vi "HFRR ADV v06.vi"() -> ()   [LabVIEW 2025] (continued)
                  n3132 = property on="Sample Temperature ( °C )" class="XYGraph (strict)"("X Scale.Name Label.Text"=w4406) -> ()  [unwired: 2 in, 2 out]
                  n3133 = property on="Coefficient Of Friction" class="XYGraph (strict)"("X Scale.Name Label.Text"=w4406) -> ()  [unwired: 2 in, 2 out]
                }
                frame 81 {
                  n3134 = property on="Air Temperature  ( °C )" class="XYGraph (strict)"("Y Scale.Name Label.Text"=w4407) -> ()  [unwired: 2 in, 2 out]
                }
                frame 82 {
                  n3135 = local write "S 84"(w4408) -> ()
                }
                frame 83 {
                  n3136 = local write "S 85"(w4409) -> ()
                }
                frame 84 {
                  n3137 = local write "S 86"(w4410) -> ()
                }
                frame 85 {
                  n3138 = local write "S 87"(w4411) -> ()
                }
                frame 86 {
                  n3139 = local write "S 88"(w4412) -> ()
                }
                frame 87 {
                  n3140 = property on="FF Calibration g" class="WFGraph (strict)"("Y Scale.Name Label.Text"=w4413) -> ()  [unwired: 2 in, 2 out]
                }
                frame 88 {
                  n3141 = local write "S 90"(w4414) -> ()
                }
                frame 89 {
                  n3142 = local write "S 91"(w4415) -> ()
                }
                frame 90 {
                  n3143 = local write "S 92"(w4416) -> ()
                }
                frame 91 {
                  n3144 = local write "S 93"(w4417) -> ()
                }
                frame 92 {
                  n3145 = local write "S 94"(w4418) -> ()
                }
                frame 93 {
                  n3146 = local write "S 95"(w4419) -> ()
                }
                frame 94 {
                  n3147 = local write "S 96"(w4420) -> ()
                }
                frame 95 {
                  n3148 = local write "S 97"(w4421) -> ()
                }
                frame 96 {
                  n3149 = local write "S 98"(w4422) -> ()
                }
                frame 97 {
                  n3150 = local write "S 99"(w4423) -> ()
                }
                frame 98 {
                  n3151 = local write "S 100"(w4424) -> ()
                }
                frame 99 {
                  n3152 = local write "S 101"(w4425) -> ()
                }
                frame 100 {
                  n3153 = local write "S 102"(w4426) -> ()
                }
                frame 101 {
                  n3154 = local write "S 103"(w4427) -> ()
                }
                frame 102 {
                  n3155 = local write "S 104"(w4428) -> ()
                }
                frame 103 {
                  n3156 = local write "S 105"(w4429) -> ()
                }
                frame 104 {
                  n3157 = local write "S 106"(w4430) -> ()
                }
                frame 105 {
                }
                frame 106 {
                  n3158 = property on="OK Button 17" class="Bool (strict)"("Boolean Text.Text"=w4431) -> ()  [unwired: 2 in, 2 out]
                }
                frame 107 {
                  n3159 = property on="OK Button 16" class="Bool (strict)"("Boolean Text.Text"=w4432) -> ()  [unwired: 2 in, 2 out]
                }
                frame 108 {
                  n3160 = property on="TITTLE" class="Str"("Caption.Text"=w4433) -> ()  [unwired: 2 in, 2 out]
                }
                frame 109 {
                  "String 30" <- w4434
                }
                frame 110 {
                  n3161 = property on="Test Date" class="Str"("Caption.Text"=w4435) -> ()  [unwired: 2 in, 2 out]
                  "String 31" <- w4435
                }
                frame 111 {
                  n3162 = property on="Sample ID" class="Str"("Caption.Text"=w4436) -> ()  [unwired: 2 in, 2 out]
                  "String 32" <- w4436
                }
                frame 112 {
                  n3163 = property on="Tested by" class="Str"("Caption.Text"=w4437) -> ()  [unwired: 2 in, 2 out]
                  "String 33" <- w4437
                }
                frame 113 {
                  n3164 = property on="System Configured Printers 2" class="Arr (strict)"("Caption.Text"=w4438) -> ()  [unwired: 2 in, 2 out]
                }
                frame 114 {
                  n3165 = property on="Selected Printer" class="Str"("Caption.Text"=w4439) -> ()  [unwired: 2 in, 2 out]
                }
                frame 115 {
                  n3166 = property on="Select Printer 3" class="DigNum (strict)"("Caption.Text"=w4440) -> ()  [unwired: 2 in, 2 out]
                }
                frame 116 {
                  n3167 = property on="Print" class="Bool (strict)"("Boolean Text.Text"=w4441) -> ()  [unwired: 2 in, 2 out]
                }
                frame 117 {
                  "String 41" <- w4442
                }
                frame 118 {
                  n3168 = property on="tested by" class="Str"("Caption.Text"=w4443) -> ()  [unwired: 2 in, 2 out]
                }
                frame 119 {
                }
                frame 120 {
                  n3169 = property on="Export" class="Bool (strict)"("Boolean Text.Text"=w4444) -> ()  [unwired: 2 in, 2 out]
                }
                frame 121 {
                  n3170 = property on="TEMP INTERCEPT:" class="DigNum (strict)"("Caption.Text"=w4445) -> ()  [unwired: 2 in, 2 out]
                }
                frame 122 {
                  n3171 = property on="AIR TEMP INTERCEPT:" class="DigNum (strict)"("Caption.Text"=w4446) -> ()  [unwired: 2 in, 2 out]
                }
                frame 123 {
                  n3172 = property on="Select File Type" class="Enum (strict)"("Caption.Text"=w4447) -> ()  [unwired: 2 in, 2 out]
                }
                frame 124 {
                  n3173 = property on="s.NO" class="Str"("Caption.Text"=w4448) -> ()  [unwired: 2 in, 2 out]
                  "String 45" <- w4448
                }
                frame 125 {
                  n3174 = property on="trip1 8" class="Bool (strict)"("Boolean Text.Text"=w4449) -> ()  [unwired: 2 in, 2 out]
                }
                frame 126, Default {
                }
              }
            }
          }
          frame #1 {
            w4457 = TRUE ("Visible")
            n3175 = local read "S 91"() -> (w4474:string)
            n3176 = local read "S 90"() -> (w4473:string)
            n3177 = local read "S 88"() -> (w4472:string)
            n3178 = property on="Threshold" class="DigNum (strict)"("Caption.Text"=w4474) -> ()  [unwired: 2 in, 2 out]
            n3179 = property on="File Path" class="Path"("Caption.Text"=w4473) -> ()  [unwired: 2 in, 2 out]
            n3180 = property on="SrvM CP" class="Bool (strict)"("Boolean Text.Text"=w4472) -> ()  [unwired: 2 in, 2 out]
            n3181 = local read "S 71"() -> (w4467:string)
            n3182 = local read "S 86"() -> (w4469:string)
            n3183 = local read "S 85"() -> (w4470:string)
            n3184 = local read "S 87"() -> (w4468:string)
            n3185 = local read "S 84"() -> (w4471:string)
            n3186 = local read "S 103"() -> (w4456:string)
            n3187 = local read "S 104"() -> (w4455:string)
            n3188 = property on="ENTER THE NEW PASSWORD" class="Str"("Caption.Text"=w4468) -> ()  [unwired: 2 in, 2 out]
            n3189 = property on="Password" class="Str"("Caption.Text"=w4470) -> ()  [unwired: 2 in, 2 out]
            n3190 = property on="ENTER CURRENT PASSWORD" class="Str"("Caption.Text"=w4469) -> ()  [unwired: 2 in, 2 out]
            n3191 = property on="EDIT" class="Bool (strict)"("Boolean Text.Text"=w4467) -> ()  [unwired: 2 in, 2 out]
            n3192 = property on="SAVE" class="Bool (strict)"("Boolean Text.Text"=w4471) -> ()  [unwired: 2 in, 2 out]
            n3193 = Build Array(w4456, w4455) -> (w4454:string[])
            n3194 = property on="Heater Button" class="Bool (strict)"("Strings [4]"=w4454) -> ()  [unwired: 2 in, 2 out]
            n3195 = property on="CH-HUMIDITY WET" class="DigNum (strict)"("Caption.Size to Text?"=w4457) -> ()  [unwired: 2 in, 2 out]
            n3196 = property on="CH-HUMIDITY DRY" class="DigNum (strict)"("Caption.Size to Text?"=w4457) -> ()  [unwired: 2 in, 2 out]
            n3197 = property on="CH-POWER -" class="DigNum (strict)"("Caption.Size to Text?"=w4457) -> ()  [unwired: 2 in, 2 out]
            n3198 = property on="CH-HEATER" class="DigNum (strict)"("Caption.Size to Text?"=w4457) -> ()  [unwired: 2 in, 2 out]
            n3199 = property on="CH-POWER +" class="DigNum (strict)"("Caption.Size to Text?"=w4457) -> ()  [unwired: 2 in, 2 out]
            n3200 = local read "S 92"() -> (w4466:string)
            n3201 = local read "S 93"() -> (w4465:string)
            n3202 = local read "S 105"() -> (w4452:string)
            n3203 = local read "S 106"() -> (w4451:string)
            n3204 = Build Array(w4466, w4465) -> ()  [unwired: 1 out]
            n3205 = Build Array(w4452, w4451) -> (w4453:string[])
            n3206 = local read "S 95"() -> (w4463:string)
            n3207 = local read "S 94"() -> (w4464:string)
            n3208 = local read "bs"() -> (w4479:string)
            n3209 = local read "as"() -> (w4480:string)
            n3210 = property on="Humidity" class="Bool (strict)"("Strings [4]"=w4453) -> ()  [unwired: 2 in, 2 out]
            n3211 = Concatenate Strings(w4479, "\r", w4480) -> ()  [unwired: 1 out]
            n3212 = property on="STROKE GAIN :" class="DigNum (strict)"("Caption.Text"=w4463) -> ()  [unwired: 2 in, 2 out]
            n3213 = property on="DISPLACEMENT :" class="DigNum (strict)"("Caption.Text"=w4464) -> ()  [unwired: 2 in, 2 out]
            n3214 = property on="Rh After" class="DigNum (strict)"("Caption.Size to Text?"=TRUE ("Caption.Size to Text")) -> ()  [unwired: 2 in, 2 out]
            n3215 = local read "S 48"() -> (w4503:string)
            n3216 = local read "S 50"() -> (w4501:string)
            n3217 = local read "S 51"() -> (w4500:string)
            n3218 = local read "S 49"() -> (w4502:string)
            n3219 = local read "S 52"() -> (w4499:string)
            n3220 = local read "as"() -> (w4484:string)
            n3221 = local read "bs"() -> (w4485:string)
            n3222 = local read "S 56"() -> (w4498:string)
            n3223 = local read "S 57"() -> (w4497:string)
            n3224 = local read "S 58"() -> (w4496:string)
            n3225 = local read "S 59"() -> (w4495:string)
            n3226 = property on="OPEN" class="Bool (strict)"("Boolean Text.Text"=w4499) -> ()  [unwired: 2 in, 2 out]
            n3227 = property on="OPEN 1" class="Bool (strict)"("Boolean Text.Text"=w4503) -> ()  [unwired: 2 in, 2 out]
            n3228 = property on="OPEN 2" class="Bool (strict)"("Boolean Text.Text"=w4502) -> ()  [unwired: 2 in, 2 out]
            n3229 = property on="OPEN 3" class="Bool (strict)"("Boolean Text.Text"=w4501) -> ()  [unwired: 2 in, 2 out]
            n3230 = property on="OPEN 4" class="Bool (strict)"("Boolean Text.Text"=w4500) -> ()  [unwired: 2 in, 2 out]
            n3231 = Concatenate Strings(w4485, "\r", w4484) -> ()  [unwired: 1 out]
            n3232 = local read "S 102"() -> (w4458:string)
            n3233 = property on="КОФ1" class="DigNum (strict)"("Caption.Text"=w4498) -> ()  [unwired: 2 in, 2 out]
            n3234 = local read "S 98"() -> (w4462:string)
            n3235 = local read "S 99"() -> (w4461:string)
            n3236 = local read "S 100"() -> (w4460:string)
            n3237 = local read "S 101"() -> (w4459:string)
            n3238 = property on="КОФ2" class="DigNum (strict)"("Caption.Text"=w4497) -> ()  [unwired: 2 in, 2 out]
            n3239 = property on="КОФ3" class="DigNum (strict)"("Caption.Text"=w4496) -> ()  [unwired: 2 in, 2 out]
            n3240 = property on="КОФ4" class="DigNum (strict)"("Caption.Text"=w4495) -> ()  [unwired: 2 in, 2 out]
            n3241 = local read "bs"() -> (w4483:string)
            n3242 = local read "as"() -> (w4482:string)
            n3243 = property on="CH-POWER +" class="DigNum (strict)"("Caption.Text"=w4462) -> ()  [unwired: 2 in, 2 out]
            n3244 = property on="CH-POWER -" class="DigNum (strict)"("Caption.Text"=w4461) -> ()  [unwired: 2 in, 2 out]
            n3245 = property on="CH-HEATER" class="DigNum (strict)"("Caption.Text"=w4460) -> ()  [unwired: 2 in, 2 out]
            n3246 = property on="CH-HUMIDITY DRY" class="DigNum (strict)"("Caption.Text"=w4459) -> ()  [unwired: 2 in, 2 out]
            n3247 = property on="CH-HUMIDITY WET" class="DigNum (strict)"("Caption.Text"=w4458) -> ()  [unwired: 2 in, 2 out]
            n3248 = local read "S 60"() -> (w4494:string)
            n3249 = local read "S 54"() -> (w4504:string)
            n3250 = Concatenate Strings(w4483, "\r", w4482) -> ()  [unwired: 1 out]
            n3251 = Concatenate Strings(w4504, w4494) -> ()  [unwired: 1 out]
            n3252 = local read "S 77"() -> (→"String 43":string)
            n3253 = local read "S 76"() -> (w4477:string)
            n3254 = local read "S 78"() -> (w4476:string)
            n3255 = local read "S 71"() -> (w4488:string)
            n3256 = local read "S 66"() -> (w4493:string)
            n3257 = local read "S 67"() -> (w4492:string)
            n3258 = local read "S 68"() -> (w4491:string)
            n3259 = local read "S 69"() -> (w4490:string)
            n3260 = local read "S 70"() -> (w4489:string)
            n3261 = property on="AIR TEMP" class="DigNum (strict)"("Caption.Text"=w4476) -> ()  [unwired: 2 in, 2 out]
            n3262 = property on="Set Strk" class="DigNum (strict)"("Caption.Text"=w4477) -> ()  [unwired: 2 in, 2 out]
            n3263 = property on="FRIC. FORCE :" class="DigNum (strict)"("Caption.Text"=w4493) -> ()  [unwired: 2 in, 2 out]
            n3264 = property on="TEMPERATURE :" class="DigNum (strict)"("Caption.Text"=w4492) -> ()  [unwired: 2 in, 2 out]
            n3265 = property on="SPEED OUT:" class="DigNum (strict)"("Caption.Text"=w4491) -> ()  [unwired: 2 in, 2 out]
            n3266 = property on="AIR TEMPERATURE :" class="DigNum (strict)"("Caption.Text"=w4490) -> ()  [unwired: 2 in, 2 out]
            n3267 = property on="HUMIDITY:" class="DigNum (strict)"("Caption.Text"=w4489) -> ()  [unwired: 2 in, 2 out]
            n3268 = property on="EDIT" class="Bool (strict)"("Boolean Text.Text"=w4488) -> ()  [unwired: 2 in, 2 out]
            n3269 = local read "S 79"() -> (w4475:string)
            n3270 = property on="Stroke" class="DigNum (strict)"("Caption.Text"=w4475) -> ()  [unwired: 2 in, 2 out]
          }
          frame #2 {
          }
        }
        n3271 = local write "Lan flag"(10.0 ("Lan flag")) -> ()
      }
      frame Enabled {
      }
    }
    n3272 = Wait (ms)(milliseconds to wait=u32 2000) -> ()  [unwired: 1 out]
    n3273 = local read "Quit"() -> (w4277:bool)
  }
  n3274 = disable-structure shown="Disabled" {
    frame Disabled {
      n3275 = while {
        tunnel: [w4506] -> _
        i -> [w4506]
        stop <- w4505 continue-if-true
        n3276 = Wait (ms)(milliseconds to wait=u32 50) -> ()  [unwired: 1 out]
        n3277 = stacked-sequence {
          frame #0 {
            # "Controls Text color"
            # "Controls BG color"
            n3278 = property on="FILE" class="Str"("Text.Text Colors:Text Color"="SC  Text") -> ()  [unwired: 2 in, 2 out]
            n3279 = property on="Fuel Discription :" class="Str"("Text.Text Colors:Text Color"="SC  Text") -> ()  [unwired: 2 in, 2 out]
            n3280 = property on="tested by" class="Str"("Text.Text Colors:Text Color"="SC  Text") -> ()  [unwired: 2 in, 2 out]
            n3281 = property on="Remarks :" class="Str"("Text.Text Colors:Text Color"="SC  Text") -> ()  [unwired: 2 in, 2 out]
            n3282 = property class="DigNum (strict)"("Numeric Text.Text Colors:BG Color"="NC BG") -> ()  [unwired: 2 in, 2 out]
            n3283 = property class="DigNum (strict)"("Numeric Text.Text Colors:BG Color"="NC BG") -> ()  [unwired: 2 in, 2 out]
            n3284 = property class="DigNum (strict)"("Numeric Text.Text Colors:BG Color"="NC BG") -> ()  [unwired: 2 in, 2 out]
            n3285 = property class="DigNum (strict)"("Numeric Text.Text Colors:BG Color"="NC BG") -> ()  [unwired: 2 in, 2 out]
            n3286 = property class="DigNum (strict)"("Numeric Text.Text Colors:BG Color"="NC BG") -> ()  [unwired: 2 in, 2 out]
            n3287 = property class="DigNum (strict)"("Numeric Text.Text Colors:BG Color"="NC BG") -> ()  [unwired: 2 in, 2 out]
            n3288 = property class="DigNum (strict)"("Numeric Text.Text Colors:BG Color"="NC BG") -> ()  [unwired: 2 in, 2 out]
            n3289 = property class="DigNum (strict)"("Numeric Text.Text Colors:BG Color"="NC BG") -> ()  [unwired: 2 in, 2 out]
            n3290 = property class="DigNum (strict)"("Numeric Text.Text Colors:BG Color"="NC BG") -> ()  [unwired: 2 in, 2 out]
            n3291 = property class="DigNum (strict)"("Numeric Text.Text Colors:BG Color"="NC BG") -> ()  [unwired: 2 in, 2 out]
            n3292 = property class="DigNum (strict)"("Numeric Text.Text Colors:BG Color"="NC BG") -> ()  [unwired: 2 in, 2 out]
            n3293 = property class="DigNum (strict)"("Numeric Text.Text Colors:BG Color"="NC BG") -> ()  [unwired: 2 in, 2 out]
            n3294 = property on="FILE" class="Str"("Text.Text Colors:BG Color"="SC BG 3") -> ()  [unwired: 2 in, 2 out]
            n3295 = property on="Fuel Discription :" class="Str"("Text.Text Colors:BG Color"="SC BG 3") -> ()  [unwired: 2 in, 2 out]
            n3296 = property on="tested by" class="Str"("Text.Text Colors:BG Color"="SC BG 3") -> ()  [unwired: 2 in, 2 out]
            n3297 = property on="Remarks :" class="Str"("Text.Text Colors:BG Color"="SC BG 3") -> ()  [unwired: 2 in, 2 out]
            n3298 = property class="DigNum (strict)"("Numeric Text.Text Colors:Text Color"="NC Text") -> ()  [unwired: 2 in, 2 out]
            n3299 = property class="DigNum (strict)"("Numeric Text.Text Colors:Text Color"="NC Text") -> ()  [unwired: 2 in, 2 out]
            n3300 = property class="DigNum (strict)"("Numeric Text.Text Colors:Text Color"="NC Text") -> ()  [unwired: 2 in, 2 out]
            n3301 = property class="DigNum (strict)"("Numeric Text.Text Colors:Text Color"="NC Text") -> ()  [unwired: 2 in, 2 out]
            n3302 = property class="DigNum (strict)"("Numeric Text.Text Colors:Text Color"="NC Text") -> ()  [unwired: 2 in, 2 out]
            n3303 = property class="DigNum (strict)"("Numeric Text.Text Colors:Text Color"="NC Text") -> ()  [unwired: 2 in, 2 out]
            n3304 = property class="DigNum (strict)"("Numeric Text.Text Colors:Text Color"="NC Text") -> ()  [unwired: 2 in, 2 out]
            n3305 = property class="DigNum (strict)"("Numeric Text.Text Colors:Text Color"="NC Text") -> ()  [unwired: 2 in, 2 out]
            n3306 = property class="DigNum (strict)"("Numeric Text.Text Colors:Text Color"="NC Text") -> ()  [unwired: 2 in, 2 out]
            n3307 = property class="DigNum (strict)"("Numeric Text.Text Colors:Text Color"="NC Text") -> ()  [unwired: 2 in, 2 out]
            n3308 = property class="DigNum (strict)"("Numeric Text.Text Colors:Text Color"="NC Text") -> ()  [unwired: 2 in, 2 out]
            n3309 = property class="DigNum (strict)"("Numeric Text.Text Colors:Text Color"="NC Text") -> ()  [unwired: 2 in, 2 out]
            n3310 = property class="DigNum (strict)"("Numeric Text.Text Colors:Text Color"="NI Text  2") -> ()  [unwired: 2 in, 2 out]
            n3311 = property class="DigNum (strict)"("Numeric Text.Text Colors:Text Color"="NI Text  2") -> ()  [unwired: 2 in, 2 out]
            n3312 = property class="DigNum (strict)"("Numeric Text.Text Colors:Text Color"="NI Text  2") -> ()  [unwired: 2 in, 2 out]
            n3313 = property class="DigNum (strict)"("Numeric Text.Text Colors:Text Color"="NI Text  2") -> ()  [unwired: 2 in, 2 out]
            n3314 = property class="DigNum (strict)"("Numeric Text.Text Colors:Text Color"="NI Text  2") -> ()  [unwired: 2 in, 2 out]
            n3315 = property class="DigNum (strict)"("Numeric Text.Text Colors:Text Color"="NI Text  2") -> ()  [unwired: 2 in, 2 out]
            n3316 = property class="DigNum (strict)"("Numeric Text.Text Colors:Text Color"="NI Text  2") -> ()  [unwired: 2 in, 2 out]
            n3317 = property class="DigNum (strict)"("Numeric Text.Text Colors:Text Color"="NI Text  2") -> ()  [unwired: 2 in, 2 out]
            n3318 = property class="DigNum (strict)"("Numeric Text.Text Colors:Text Color"="NI Text  2") -> ()  [unwired: 2 in, 2 out]
            n3319 = property class="DigNum (strict)"("Numeric Text.Text Colors:Text Color"="NI Text  2") -> ()  [unwired: 2 in, 2 out]
            n3320 = property class="DigNum (strict)"("Numeric Text.Text Colors:Text Color"="NI Text  2") -> ()  [unwired: 2 in, 2 out]
            n3321 = property class="DigNum (strict)"("Numeric Text.Text Colors:Text Color"="NI Text  2") -> ()  [unwired: 2 in, 2 out]
            n3322 = property class="DigNum (strict)"("Numeric Text.Text Colors:Text Color"="NI Text  2") -> ()  [unwired: 2 in, 2 out]
            n3323 = property class="DigNum (strict)"("Numeric Text.Text Colors:Text Color"="NI Text  2") -> ()  [unwired: 2 in, 2 out]
            n3324 = property class="DigNum (strict)"("Numeric Text.Text Colors:Text Color"="NI Text  2") -> ()  [unwired: 2 in, 2 out]
            n3325 = property class="DigNum (strict)"("Numeric Text.Text Colors:Text Color"="NI Text  2") -> ()  [unwired: 2 in, 2 out]
            n3326 = property on="Coefficient Of Friction" class="XYGraph (strict)"("Plot Area:Colors:FG Color"="GFG  2", "Plot Area:Colors:BG Color"="GBG   2") -> ()  [unwired: 2 in, 2 out]
            n3327 = property on="Humidity ( %Rh )" class="XYGraph (strict)"("Plot Area:Colors:FG Color"="GFG  2", "Plot Area:Colors:BG Color"="GBG   2") -> ()  [unwired: 2 in, 2 out]
            n3328 = property on="Air Temperature  ( °C )" class="XYGraph (strict)"("Plot Area:Colors:FG Color"="GFG  2", "Plot Area:Colors:BG Color"="GBG   2") -> ()  [unwired: 2 in, 2 out]
            n3329 = property on="Sample Temperature ( °C )" class="XYGraph (strict)"("Plot Area:Colors:FG Color"="GFG  2", "Plot Area:Colors:BG Color"="GBG   2") -> ()  [unwired: 2 in, 2 out]
            n3330 = property class="DigNum (strict)"("Numeric Text.Text Colors:BG Color"="NI BG 2") -> ()  [unwired: 2 in, 2 out]
            n3331 = property class="DigNum (strict)"("Numeric Text.Text Colors:BG Color"="NI BG 2") -> ()  [unwired: 2 in, 2 out]
            n3332 = property class="DigNum (strict)"("Numeric Text.Text Colors:BG Color"="NI BG 2") -> ()  [unwired: 2 in, 2 out]
            n3333 = property class="DigNum (strict)"("Numeric Text.Text Colors:BG Color"="NI BG 2") -> ()  [unwired: 2 in, 2 out]
            n3334 = property class="DigNum (strict)"("Numeric Text.Text Colors:BG Color"="NI BG 2") -> ()  [unwired: 2 in, 2 out]
            n3335 = property class="DigNum (strict)"("Numeric Text.Text Colors:BG Color"="NI BG 2") -> ()  [unwired: 2 in, 2 out]
            n3336 = property class="DigNum (strict)"("Numeric Text.Text Colors:BG Color"="NI BG 2") -> ()  [unwired: 2 in, 2 out]
            n3337 = property class="DigNum (strict)"("Numeric Text.Text Colors:BG Color"="NI BG 2") -> ()  [unwired: 2 in, 2 out]
            n3338 = property class="DigNum (strict)"("Numeric Text.Text Colors:BG Color"="NI BG 2") -> ()  [unwired: 2 in, 2 out]
            n3339 = property class="DigNum (strict)"("Numeric Text.Text Colors:BG Color"="NI BG 2") -> ()  [unwired: 2 in, 2 out]
            n3340 = property class="DigNum (strict)"("Numeric Text.Text Colors:BG Color"="NI BG 2") -> ()  [unwired: 2 in, 2 out]
            n3341 = property class="DigNum (strict)"("Numeric Text.Text Colors:BG Color"="NI BG 2") -> ()  [unwired: 2 in, 2 out]
            n3342 = property class="DigNum (strict)"("Numeric Text.Text Colors:BG Color"="NI BG 2") -> ()  [unwired: 2 in, 2 out]
            n3343 = property class="DigNum (strict)"("Numeric Text.Text Colors:BG Color"="NI BG 2") -> ()  [unwired: 2 in, 2 out]
            n3344 = property class="DigNum (strict)"("Numeric Text.Text Colors:BG Color"="NI BG 2") -> ()  [unwired: 2 in, 2 out]
            n3345 = property class="DigNum (strict)"("Numeric Text.Text Colors:BG Color"="NI BG 2") -> ()  [unwired: 2 in, 2 out]
            n3346 = property class="Bool"("Colors [4]"="Boolean BC T & BG") -> ()  [unwired: 2 in, 2 out]
            n3347 = property on="Save & Continue" class="Bool (strict)"("Colors [4]"="Boolean BC T & BG") -> ()  [unwired: 2 in, 2 out]
            n3348 = property on="Heater Button" class="Bool (strict)"("Colors [4]"="Boolean BC T & BG") -> ()  [unwired: 2 in, 2 out]
            n3349 = property class="Bool"("Colors [4]"="Boolean BC T & BG") -> ()  [unwired: 2 in, 2 out]
            n3350 = property on="Humidity" class="Bool (strict)"("Colors [4]"="Boolean BC T & BG") -> ()  [unwired: 2 in, 2 out]
            n3351 = property class="Bool (strict)"("Colors [4]"="Boolean BC T & BG") -> ()  [unwired: 2 in, 2 out]
            n3352 = property on="RUN" class="Bool (strict)"("Colors [4]"="Boolean BC T & BG") -> ()  [unwired: 2 in, 2 out]
            n3353 = property on="trip1 8" class="Bool (strict)"("Colors [4]"="Boolean BC T & BG") -> ()  [unwired: 2 in, 2 out]
            n3354 = property class="Bool"("Colors [4]"="Boolean BC T & BG") -> ()  [unwired: 2 in, 2 out]
            n3355 = property class="Bool (strict)"("Colors [4]"="Boolean BC T & BG") -> ()  [unwired: 2 in, 2 out]
            n3356 = property on="OPEN 1" class="Bool (strict)"("Colors [4]"="Boolean BC T & BG 2") -> ()  [unwired: 2 in, 2 out]
            n3357 = property on="OPEN 2" class="Bool (strict)"("Colors [4]"="Boolean BC T & BG 2") -> ()  [unwired: 2 in, 2 out]
            n3358 = property on="OPEN 3" class="Bool (strict)"("Colors [4]"="Boolean BC T & BG 2") -> ()  [unwired: 2 in, 2 out]
            n3359 = property on="OPEN 4" class="Bool (strict)"("Colors [4]"="Boolean BC T & BG 2") -> ()  [unwired: 2 in, 2 out]
            n3360 = property on="OPEN" class="Bool (strict)"("Colors [4]"="Boolean BC T & BG 2") -> ()  [unwired: 2 in, 2 out]
            n3361 = property on="rstv2" class="Bool"("Colors [4]"="Boolean BC T & BG 2") -> ()  [unwired: 2 in, 2 out]
            n3362 = property on="RST CP" class="Bool"("Colors [4]"="Boolean BC T & BG 2") -> ()  [unwired: 2 in, 2 out]
            n3363 = property on="RSTV1 3" class="Bool"("Colors [4]"="Boolean BC T & BG 2") -> ()  [unwired: 2 in, 2 out]
            n3364 = property on="RSTV1 2" class="Bool"("Colors [4]"="Boolean BC T & BG 2") -> ()  [unwired: 2 in, 2 out]
          }
          frame #1 {
          }
        }
        n3365 = local read "Quit"() -> (w4505:bool)
      }
    }
    frame Enabled {
    }
  }
  n3366 = while {
    shift-right: [w4523] -> _
    shift-left: _ -> [w4524]
    shift-right: [w4521] -> _
    shift-left: T13 {"Read Heave and Surge"="", "Bytes at Heave Port"=0.0, "Heave and Surge COM Port:"="COM9", "Com Port 2"="COM7", "Residual Due"="", "Heave COM Status 2"=TRUE, "Heave COM Status"=TRUE, "Port 2"=TRUE, "Sway PPR"=6400.0, "Surge PPR"=6400.0, "Heave PPR"=6400.0, "Sway Pitch"=2.0, "Surge Pitch"=3.0, "Heave Pitch"=4.0, "Sway Pulses/mm"=320.0, "Surge Pulses/mm"=1600.0, "Heave Pulses/mm"=1600.0, "inner loop"=0.0, "Read Heave and Surge 2"="", "String 36"="", "Write S"=FALSE, "WriteCC1"=[""], "Heave COM Loop"=0, "LastCom"="", "EXIT"=FALSE, "Error Heave"={"status"=TRUE, "code"=-1073807343, "source"=""}} -> [w4520]
    shift-right: [w4518] -> _
    shift-left: enum16{"init", "MAIN", "Panel Close"}."init" -> [w4519]
    stop <- w4522 stop-if-true
    n3367 = case shown="\"MAIN\"" w4519 {
      tunnel: w4524 -> [w4538 w4553 w4623 w4625]
      tunnel: [w4532 w4571 w4623 w4625] -> w4523
      tunnel: [_ _ TRUE _] -> w4522
      tunnel: [w4528 w4568 w4621 w4624] -> w4521
      tunnel: w4520 -> [w4535 w4552 w4621 w4624]
      tunnel: [enum16{"init", "MAIN", "Panel Close"}."MAIN" w4546 _ _] -> w4518
      frame "init" {
        n3368 = Bundle By Name(cluster=w4535, "Heave and Surge COM Port:"="Humidity :") -> (w4534:T13)
        n3369 = call "Instrument fgv.vi"("Enum"=T22."INIT", "error in (no error) 2"=w4538, "INPUT"=w4534) -> ("error"=w4536:errorcluster, "output"=w4531:T13)  [unwired: 6 in, 1 out]
        n3370 = case shown="No Error" w4536 {
          selector: w4536 -> [w4540 _]
          tunnel: [w4540 w4544] -> w4532
          tunnel: w4531 -> [w4539 w4542]
          tunnel: [w4539 w4541] -> w4529
          frame No Error {
          }
          frame Error {
            n3371 = call "Instrument fgv.vi"("Enum"=T22."ERROR INIT", "INPUT"=w4542) -> ("error"=w4545:errorcluster, "output"=w4541:T13)  [unwired: 7 in, 1 out]
            n3372 = call <vilib>:"Clear Errors.vi"("error in (no error)"=w4545) -> ("error out"=w4544:errorcluster)  [unwired: 5 in, 1 out]
          }
        }
        n3373 = local read "LastCom"() -> (w4527:string)
        n3374 = Unbundle By Name(w4529) -> ("Heave COM Status 2"=→"Heave COM Status 2" →"Instrument Status":bool, "Error Heave"=→"Error Heave":errorcluster)  [unwired: 1 out]
        n3375 = Bundle By Name(cluster=w4529, "LastCom"=w4527) -> (w4528:T13)
      }
      frame "MAIN" {
        n3376 = Unbundle By Name(w4552) -> ("Com Port 2"=w4573:refnum<visa-resource-name>)
        n3377 = local write "Com Port 4"(w4573) -> ()
        n3378 = local read "Humidity :"() -> (w4550:refnum<visa-resource-name>)
        n3379 = Divide(x="Heave PPR", y="Heave Pitch") -> (x/y=→"Heave Pulses/mm":dbl)
        n3380 = Bundle By Name(cluster=w4552, "Heave and Surge COM Port:"=w4550) -> (w4551:T13)
        n3381 = Equal?(x=w4573, y=w4550) -> (x = y?=w4572:bool)
        n3382 = Divide(x="Sway PPR", y="Sway Pitch") -> (x/y=→"Sway Pulses/mm":dbl)
        n3383 = case shown="True" w4572 {
          tunnel: [w4577 w4594] -> w4571
          tunnel: w4553 -> [w4578 w4600]
          tunnel: w4551 -> [w4576 w4598]
          tunnel: [w4575 w4593] -> w4568
          frame False {
            n3384 = call <vilib>:"Clear Errors.vi"("error in (no error)"=w4578) -> ("error out"=w4574:errorcluster)  [unwired: 5 in, 1 out]
            n3385 = call "Instrument fgv.vi"("Enum"=T22."ERROR INIT", "error in (no error) 2"=w4574, "INPUT"=w4576) -> ("error"=w4580:errorcluster, "output"=w4575:T13)  [unwired: 6 in, 1 out]
            n3386 = call <vilib>:"Clear Errors.vi"("error in (no error)"=w4580) -> ("error out"=w4577:errorcluster)  [unwired: 5 in, 1 out]
          }
          frame True {
            n3387 = call "Instrument fgv.vi"("Enum"=T22."READ", "error in (no error) 2"=w4600, "INPUT"=w4598) -> ("error"=w4599:errorcluster, "output"=w4590:T13)  [unwired: 6 in, 1 out]
            n3388 = Bundle By Name(cluster=w4590, "String 36"="String") -> (w4589:T13)
            n3389 = case shown="True" "Write S" {
              selector: "Write S" -> [_ w4620]
              tunnel: w4599 -> [w4613 w4619]
              tunnel: [w4613 w4618] -> w4586
              tunnel: w4589 -> [w4612 w4615]
              tunnel: [w4612 w4614] -> w4585
              frame False {
              }
              frame True {
                n3390 = Not(x=w4620) -> (.not. x?=w4616:bool)
                n3391 = local write "Write S"(w4616) -> ()
                n3392 = call "Instrument fgv.vi"("Enum"=T22."MANUAL WRITE", "error in (no error) 2"=w4619, "INPUT"=w4615) -> ("error"=w4618:errorcluster, "output"=w4614:T13)  [unwired: 6 in, 1 out]
              }
            }
            n3393 = Array Size(array="WriteHumidity") -> (size(s)=w4583:i32)
            n3394 = Greater Than 0?(x=w4583) -> (x > 0?=w4581:bool)
            n3395 = call "Instrument fgv.vi"("Enum"=T22."WRITE", "error in (no error) 2"=w4586, "WriteCC1"="WriteHumidity", "INPUT"=w4585) -> ("error"=w4596:errorcluster, "WriteCC1 2"=w4584:string[], "output"=w4595:T13)  [unwired: 5 in]
            n3396 = case shown="True" w4581 {
              tunnel: w4584 -> [_ w4602]
              frame False {
              }
              frame True {
                n3397 = local write "WriteHumidity"(w4602) -> ()
              }
            }
            n3398 = case shown="Error" w4596 {
              selector: w4596 -> [w4603 w4606]
              tunnel: w4595 -> [w4604 w4611]
              tunnel: [w4604 w4610] -> w4593
              tunnel: [w4603 w4608] -> w4594
              frame No Error {
              }
              frame Error {
                n3399 = call <vilib>:"Clear Errors.vi"("error in (no error)"=w4606) -> ("error out"=w4605:errorcluster)  [unwired: 5 in, 1 out]
                n3400 = call "Instrument fgv.vi"("Enum"=T22."ERROR INIT", "error in (no error) 2"=w4605, "INPUT"=w4611) -> ("error"=w4609:errorcluster, "output"=w4610:T13)  [unwired: 6 in, 1 out]
                n3401 = call <vilib>:"Clear Errors.vi"("error in (no error)"=w4609) -> ("error out"=w4608:errorcluster)  [unwired: 5 in, 1 out]
              }
            }
            n3402 = Unbundle By Name(w4593) -> ("LastCom"=→"LastCom":string, "Read Heave and Surge"=→"Read Humidity":string)
          }
        }
        n3403 = Divide(x="Surge PPR", y="Surge Pitch") -> (x/y=→"Surge Pulses/mm":dbl)
        n3404 = Unbundle By Name(w4568) -> ("Heave COM Status 2"=w4570:bool, "Heave COM Status"=w4569:bool, "Error Heave"=w4566:errorcluster, "Bytes at Heave Port"=→"Bytes at Humidity Port":dbl)
        n3405 = Unbundle By Name(w4566) -> ("status"=→"Humidity Port":bool)
        n3406 = local write "Error Heave"(w4566) -> ()
        n3407 = Not(x=w4569) -> (.not. x?=w4554:bool)
        n3408 = Not(x=w4570) -> (.not. x?=w4555:bool)
        n3409 = local write "Heave COM Status 2"(w4555) -> ()
        n3410 = local write "Instrument Status"(w4554) -> ()
        n3411 = local read "Quit"() -> (w4547:bool)
        n3412 = Select(t=enum16{"init", "MAIN", "Panel Close"}."Panel Close", s=w4547, f=enum16{"init", "MAIN", "Panel Close"}."MAIN") -> (s? t:f=w4546:enum16{"init", "MAIN", "Panel Close"})
      }
      frame "Panel Close" {
      }
      frame Default {
      }
    }
  }
  n3413 = while {
    stop <- w4651 stop-if-true
    n3414 = local read "Read Humidity"() -> (w4632:string)
    n3415 = call <vilib>:"High Resolution Polling Wait.vi"("seconds to wait"=0.1) -> ()  [unwired: 10 in, 1 out]
    n3416 = Spreadsheet String To Array(delimiter (Tab)=",", format string="", spreadsheet string=w4632, array type (2D Dbl)=string[] []) -> (array=w4646:string[])
    n3417 = for {
      tunnel: w4646 -> [w4656] mode=indexing
      tunnel: string[] ["STATE;", "SET;", "RH;", "T;", "AMB_RH;", "AMB_T;", "PUMP;", "FAN_IN;", "FAN_OUT;", "DEHUM;", "CURRENT;", "STALL;"] -> [w4655] mode=indexing
      tunnel: [w4654] -> w4645 mode=indexing
      n3418 = Match Pattern(string=w4656, regular expression=w4655) -> (after substring=w4654:string)  [unwired: 1 in, 3 out]
    }
    n3419 = Index Array(array=w4645) -> (element #1=→"STATE :":string, element #2=→"SET :":string, element #3=w4634:string, element #4=→"T :":string, element #5=w4631:string, element #6=→"AMB_T :":string, element #7=→"PUMP :":string, element #8=→"FAN_IN :":string, element #9=→"FAN_OUT :":string, element #10=→"DEHUM :":string, element #11=→"CURRENT :":string, element #12=→"STALL :":string)  [unwired: 12 in]
    "RH :" <- w4634
    "AMB_RH :" <- w4631
    n3420 = Fract/Exp String To Number(string=w4634) -> (number=w4626:dbl)  [unwired: 3 in, 1 out]
    n3421 = Fract/Exp String To Number(string=w4631) -> (number=w4630:dbl)  [unwired: 3 in, 1 out]
    n3422 = local write "Ambient Humidity :"(w4630) -> ()
    n3423 = Equal?(x=w4626, y=0.0) -> (x = y?=w4628:bool)
    n3424 = case shown="True" w4628 {
      tunnel: [w4652 w4653] -> w4627
      tunnel: w4626 -> [w4652 _]
      frame False {
        (unwired) 0.0
        "Humidity temp" <- w4652
      }
      frame True {
        n3425 = local read "Humidity temp"() -> (w4653:dbl)
      }
    }
    "RH Numeric:" <- w4627
    n3426 = local read "Quit"() -> (w4651:bool)
  }
  n3427 = disable-structure shown="Disabled" {
    frame Disabled {
      n3428 = while {
        tunnel: [w4890] -> _
        i -> [w4890]
        stop <- w4887 stop-if-true
        n3429 = local read "powstat"() -> (w4888:bool)
        n3430 = case shown="True" w4888 {
          frame False {
          }
          frame True {
            n3431 = local read "RUN"() -> (w4891:bool)
            n3432 = case shown="True" w4891 {
              frame False {
                w4921 = 65.0 ("y")
                n3433 = local read "Set Hz"() -> (w4949:dbl)
                n3434 = local read "NORMAL LOAD"() -> (w4950:dbl)
                n3435 = Multiply(x=w4949, y=60.0) -> (x*y=w4956:dbl)
                n3436 = Multiply(x=1.2 ("y"), y=0.949) -> (x*y=w4925:dbl)
                n3437 = Multiply(x=1.2 ("y"), y=0.8166) -> (x*y=w4929:dbl)
                n3438 = Multiply(x=1.2 ("y"), y=0.851) -> (x*y=w4924:dbl)
                n3439 = local read "FF 2"() -> (w4948:dbl)
                n3440 = Absolute Value(x=w4956) -> (abs(x)=w4954:dbl)
                n3441 = local read "Stroke"() -> (w4923:dbl)
                n3442 = Less?(x=w4923, y=w4929) -> (x < y?=w4926:bool)
                n3443 = In Range and Coerce(upper limit=w4925, x=w4923, lower limit=w4924) -> (In Range?=w4927:bool)  [unwired: 1 out]
                n3444 = case shown="13.." w4948 {
                  tunnel: [1 2 3] -> w4946
                  frame 0..10, Default {
                    # "Normal"
                  }
                  frame 11, 12 {
                  }
                  frame 13.. {
                  }
                }
                "FF STATE" <- w4946
                n3445 = local read "TEMP"() -> (w4909:dbl)
                n3446 = case shown="3601.." w4954 {
                  tunnel: [1 2 3] -> w4952
                  frame 0..3000, Default {
                    # "Normal"
                  }
                  frame 3001..3600 {
                  }
                  frame 3601.. {
                  }
                }
                n3447 = case shown="11.." w4950 {
                  tunnel: [1 3] -> w4951
                  frame 1..10, Default {
                  }
                  frame 11.. {
                  }
                }
                "NL STATE" <- w4951
                n3448 = Multiply(x=1.2 ("y"), y=0.95) -> (x*y=w4939:dbl)
                n3449 = Multiply(x=w4921, y=0.954) -> (x*y=w4913:dbl)
                n3450 = Or(x=w4926, y=w4927) -> (x .or. y?=w4928:bool)
                n3451 = Greater Or Equal?(x=w4923, y=w4939) -> (x >= y?=w4936:bool)
                n3452 = Multiply(x=w4921, y=0.99) -> (x*y=w4910:dbl)
                n3453 = Greater Or Equal?(x=w4909, y=w4910) -> (x >= y?=w4915:bool)
                n3454 = Greater Or Equal?(x=w4909, y=w4913) -> (x >= y?=w4912:bool)
                n3455 = case shown="0, 1, Default" w4923 {
                  tunnel: [1 3] -> w4940
                  frame 0, 1, Default {
                  }
                  frame 2.. {
                  }
                }
                n3456 = case shown="True" w4936 {
                  tunnel: [1 3] -> w4941
                  frame False {
                  }
                  frame True {
                  }
                }
                n3457 = case shown="True" w4928 {
                  tunnel: [1 2] -> w4942
                  frame False {
                  }
                  frame True {
                  }
                }
                n3458 = case shown="..0" w4909 {
                  tunnel: [2 3 3 1] -> w4916
                  frame 61, 62 {
                  }
                  frame 63.. {
                  }
                  frame ..0 {
                  }
                  frame 10..60, Default {
                  }
                }
                n3459 = case shown="True" w4915 {
                  tunnel: [1 3] -> w4917
                  frame False {
                  }
                  frame True {
                  }
                }
                n3460 = Number To Decimal String(number=w4952) -> (decimal integer string=w4953:string)  [unwired: 1 in]
                n3461 = case shown="True" w4912 {
                  tunnel: [1 2] -> w4918
                  frame False {
                  }
                  frame True {
                  }
                }
                n3462 = Number To Decimal String(number=1) -> (decimal integer string=→"Air temp":string)  [unwired: 1 in]
                n3463 = Number To Decimal String(number=w4946) -> (decimal integer string=→"ff_st":string)  [unwired: 1 in]
                n3464 = local write "sp_st"(w4953) -> ()
                n3465 = Number To Decimal String(number=w4951) -> (decimal integer string=→"nl_st":string)  [unwired: 1 in]
                n3466 = Build Array(w4916, w4917, w4918) -> (w4919:i32[])
                n3467 = Build Array(w4940, w4941, w4942) -> (w4943:i32[])
                n3468 = Array Max & Min(array=w4919) -> (max value=w4920:i32)  [unwired: 3 out]
                n3469 = Array Max & Min(array=w4943) -> (max value=w4944:i32)  [unwired: 3 out]
                n3470 = Number To Decimal String(number=w4920) -> (decimal integer string=w4908:string)  [unwired: 1 in]
                n3471 = Number To Decimal String(number=w4944) -> (decimal integer string=→"Stroke Ln 2":string)  [unwired: 1 in]
                n3472 = local write "temp_st"(w4908) -> ()
              }
              frame True {
                w5006 = 65.0 ("y")
                # "Healthy -1\nWarning -2\nError -3"
                n3473 = local read "TEMP"() -> (w5017:dbl)
                n3474 = local read "NORMAL LOAD"() -> (w5021:dbl)
                n3475 = local read "Set Hz"() -> (w5019:dbl)
                n3476 = Multiply(x=1.2 ("y"), y=0.949) -> (x*y=w5001:dbl)
                n3477 = Multiply(x=1.2 ("y"), y=0.8166) -> (x*y=w4997:dbl)
                n3478 = Multiply(x=1.2 ("y"), y=0.851) -> (x*y=w5002:dbl)
                n3479 = Multiply(x=w5006, y=0.954) -> (x*y=w5013:dbl)
                n3480 = Multiply(x=w5006, y=0.99) -> (x*y=w5016:dbl)
                n3481 = Greater Or Equal?(x=w5017, y=w5016) -> (x >= y?=w5011:bool)
                n3482 = Multiply(x=w5019, y=60.0) -> (x*y=w5025:dbl)
                n3483 = Greater Or Equal?(x=w5017, y=w5013) -> (x >= y?=w5014:bool)
                n3484 = local read "FF 2"() -> (w5020:dbl)
                n3485 = local read "Stroke"() -> (w5003:dbl)
                n3486 = Less?(x=w5003, y=w4997) -> (x < y?=w5000:bool)
                n3487 = In Range and Coerce(upper limit=w5001, x=w5003, lower limit=w5002) -> (In Range?=w4999:bool)  [unwired: 1 out]
                n3488 = Absolute Value(x=w5025) -> (abs(x)=w5023:dbl)
                n3489 = case shown="63.." w5017 {
                  tunnel: [2 3 3 1] -> w5010
                  frame 61, 62 {
                  }
                  frame 63.. {
                  }
                  frame ..0 {
                  }
                  frame 10..60, Default {
                  }
                }
                n3490 = case shown="True" w5011 {
                  tunnel: [1 3] -> w5009
                  frame False {
                  }
                  frame True {
                  }
                }
                n3491 = case shown="True" w5014 {
                  tunnel: [1 2] -> w5008
                  frame False {
                  }
                  frame True {
                  }
                }
                n3492 = Multiply(x=1.2 ("y"), y=0.95) -> (x*y=w4987:dbl)
                n3493 = case shown="1..10, Default" w5021 {
                  tunnel: [1 3] -> w5028
                  frame 1..10, Default {
                  }
                  frame 11.. {
                  }
                }
                n3494 = case shown="0..10, Default" w5020 {
                  tunnel: [1 2 3] -> w5027
                  frame 0..10, Default {
                  }
                  frame 11, 12 {
                  }
                  frame 13.. {
                  }
                }
                n3495 = case shown="3601.." w5023 {
                  tunnel: [1 2 3] -> w5022
                  frame 0..3000, Default {
                    # "Normal"
                  }
                  frame 3001..3600 {
                  }
                  frame 3601.. {
                  }
                }
                n3496 = Or(x=w5000, y=w4999) -> (x .or. y?=w4998:bool)
                n3497 = Greater Or Equal?(x=w5003, y=w4987) -> (x >= y?=w4990:bool)
                n3498 = case shown="0, 1, Default" w5003 {
                  tunnel: [1 3] -> w4986
                  frame 0, 1, Default {
                  }
                  frame 2.. {
                  }
                }
                n3499 = case shown="True" w4990 {
                  tunnel: [1 3] -> w4985
                  frame False {
                  }
                  frame True {
                  }
                }
                n3500 = case shown="True" w4998 {
                  tunnel: [1 2] -> w4984
                  frame False {
                  }
                  frame True {
                  }
                }
                n3501 = Build Array(w5010, w5009, w5008) -> (w5007:i32[])
                n3502 = Number To Decimal String(number=w5022) -> (decimal integer string=→"sp_st":string)  [unwired: 1 in]
                n3503 = Array Max & Min(array=w5007) -> (max value=w5004:i32)  [unwired: 3 out]
                "TEMP STATE" <- w5004
                n3504 = Number To Decimal String(number=w5028) -> (decimal integer string=w5031:string)  [unwired: 1 in]
                n3505 = Number To Decimal String(number=w5027) -> (decimal integer string=w5029:string)  [unwired: 1 in]
                n3506 = Number To Decimal String(number=w5004) -> (decimal integer string=→"temp_st":string)  [unwired: 1 in]
                n3507 = Build Array(w4986, w4985, w4984) -> (w4983:i32[])
                n3508 = local write "nl_st"(w5031) -> ()
                n3509 = local write "ff_st"(w5029) -> ()
                n3510 = Number To Decimal String(number=1) -> (decimal integer string=w5026:string)  [unwired: 1 in]
                n3511 = Array Max & Min(array=w4983) -> (max value=w4982:i32)  [unwired: 3 out]
                n3512 = local write "Air temp"(w5026) -> ()
                n3513 = Number To Decimal String(number=w4982) -> (decimal integer string=w4981:string)  [unwired: 1 in]
                n3514 = local write "Stroke Ln 2"(w4981) -> ()
              }
            }
            n3515 = local read "Stroke Ln 2"() -> (w4893:string)
            n3516 = local read "nl_st"() -> (w4899:string)
            n3517 = local read "ff_st"() -> (w4896:string)
            n3518 = local read "sp_st"() -> (w4897:string)
            n3519 = local read "temp_st"() -> (w4898:string)
            n3520 = local read "Air temp"() -> (w4892:string)
            n3521 = Replace Array Subset(array="in", new element #1=w4899, index #1=1 ("index"), new element #2=w4896, index #2=2 ("index"), new element #3=w4898, index #3=3 ("index"), new element #4=w4897, index #4=4 ("index"), new element #5=w4893, index #5=5 ("index"), new element #6=w4892, index #6=6 ("index"), new element #7="Sensor State" ("new element/subarray"), index #7=0 ("index")) -> (→"out":string[])
          }
        }
        n3522 = Wait (ms)(milliseconds to wait=u32 10) -> ()  [unwired: 1 out]
        n3523 = local read "Quit"() -> (w4887:bool)
      }
      n3524 = while {
        stop <- w4862 stop-if-true
        n3525 = local read "run replace"() -> (w4864:bool)
        n3526 = Wait (ms)(milliseconds to wait=u32 100) -> ()  [unwired: 1 out]
        n3527 = Equal?(x="FLAG 2", y=0.0) -> (x = y?=w4865:bool)
        n3528 = case shown="True" w4865 {
          frame False {
          }
          frame True {
            n3529 = local write "FLAG 2"(100.0 ("FLAG 2")) -> ()
            n3530 = call <vilib>:"Read Characters From File.vi"("file path (dialog if empty)"=path "C:/LAB-IQ-NXT/WO 2449 TT.sig", "convert eol? (no:F)"=FALSE ("append to file? (new file:F)")) -> ("character string"=w4868:string)  [unwired: 4 in, 3 out]
            n3531 = call <vilib>:"Read Characters From File.vi"("file path (dialog if empty)"=path "C:/LAB-IQ-NXT/WO 2449 TRH.sig", "convert eol? (no:F)"=FALSE ("append to file? (new file:F)")) -> ("character string"=w4869:string)  [unwired: 4 in, 3 out]
            n3532 = Decimal String To Number(string=w4868) -> (number=w4870:i32)  [unwired: 2 in, 1 out]
            n3533 = local write "Total No. of Tests"(w4870) -> ()
            n3534 = Decimal String To Number(string=w4869) -> (number=w4873:i32)  [unwired: 2 in, 1 out]
            n3535 = local write "SEN.RUN HRS"(w4873) -> ()
          }
        }
        n3536 = case shown="True" w4864 {
          frame False {
          }
          frame True {
            n3537 = Equal?(x="FLAG 4", y=0.0) -> (x = y?=w4877:bool)
            n3538 = case shown="False" w4877 {
              frame False {
                n3539 = Get Date/Time In Seconds() -> (seconds since 1Jan1904=w4883:timestamp)
                n3540 = local read "START 3"() -> (w4881:dbl)
                n3541 = To Double Precision Float(number=w4883) -> (double precision float=w4882:dbl)
                n3542 = Subtract(x=w4882, y=w4881) -> (x-y=→"SENSOR TIME":dbl)
              }
              frame True {
                n3543 = Get Date/Time In Seconds() -> (seconds since 1Jan1904=w4885:timestamp)
                n3544 = local write "FLAG 4"(100.0 ("FLAG")) -> ()
                n3545 = To Double Precision Float(number=w4885) -> (double precision float=→"START 3":dbl)
              }
            }
          }
        }
        n3546 = local read "Quit"() -> (w4862:bool)
      }
      n3547 = while {
        shift-right: [w4662] -> _
        shift-left: _ -> [w4663]
        tunnel: [w4658] -> _
        i -> [w4658]
        stop <- w4657 stop-if-true
        n3548 = Wait (ms)(milliseconds to wait=u32 50 ("Refresh Rate (ms)")) -> ()  [unwired: 1 out]
        n3549 = local read "Json End Flg"() -> (w4659:bool)
        n3550 = Not(x="Upld AR 2") -> ()  [unwired: 1 out]
        n3551 = local read "Upld AR 2"() -> (w4660:bool)
        n3552 = call "Elapsed Time9"("Time Target (s)"="Sen.Upload Rate (s)", "Reset"=FALSE, "Auto Reset"=TRUE) -> ("Time has Elapsed"=w4669:bool)  [unwired: 9 in, 7 out]
        n3553 = Or(x=w4669, y=w4659) -> (x .or. y?=w4665:bool)
        n3554 = case shown="True" w4665 {
          frame False {
          }
          frame True {
            w4761 = "\"SensorName\":\"" ("string")
            w4731 = " \"},{"
            w4756 = "\",\"SensorState\":\""
            w4758 = "\",\"SensorModelNumber\":\"" ("string")
            w4757 = "\",\"SensorRuntimeHours\":\"" ("string")
            n3555 = local read "model num"() -> (w4755:string[])
            n3556 = local read "Sensor name"() -> (w4774:string[])
            n3557 = local read "run"() -> (w4745:string[])
            n3558 = local read "SENSOR TIME"() -> (w4701:dbl)
            n3559 = local read "out"() -> (w4694:string[])
            n3560 = local read "Total No. of Tests"() -> (w4699:dbl)
            n3561 = Select(t=60.0, s="Run test 3", f=3600.0) -> (s? t:f=w4709:dbl)
            n3562 = Index Array(array=w4755, index #1=1 ("index")) -> (element #1=w4754:string, element #2=w4753:string, element #3=w4752:string, element #4=w4751:string, element #5=w4750:string, element #6=w4749:string)  [unwired: 5 in]
            n3563 = Index Array(array=w4745, index #1=1 ("index")) -> (element #1=w4744:string, element #2=w4743:string, element #3=w4742:string, element #4=w4741:string, element #5=w4740:string, element #6=w4739:string)  [unwired: 5 in]
            n3564 = Index Array(array=w4774, index #1=1 ("index")) -> (element #1=w4773:string, element #2=w4772:string, element #3=w4771:string, element #4=w4770:string, element #5=w4760:string, element #6=w4759:string)  [unwired: 5 in]
            n3565 = Index Array(array=w4694, index #1=1 ("index")) -> (element #1=w4726:string, element #2=w4725:string, element #3=w4724:string, element #4=w4723:string, element #5=w4722:string, element #6=w4721:string)  [unwired: 5 in]
            n3566 = local read "SEN.RUN HRS"() -> (w4697:dbl)
            n3567 = Divide(x=w4701, y=w4709) -> (x/y=w4708:dbl)
            n3568 = Increment(x=w4708) -> (x+1=w4704:dbl)
            n3569 = Number To Decimal String(number=w4704) -> (decimal integer string=→"run hrs":string)  [unwired: 1 in]
            n3570 = Divide(x=w4697, y=3600.0 ("f")) -> (x/y=w4692:dbl)
            n3571 = Round To Nearest(number=w4692) -> (nearest integer value=w4690:dbl)
            n3572 = Number To Decimal String(number=w4690) -> (decimal integer string=w4691:string)  [unwired: 1 in]
            n3573 = Number To Decimal String(number=w4699) -> (decimal integer string=w4700:string)  [unwired: 1 in]
            n3574 = local read "Model No"() -> (w4705:string)
            n3575 = local read "UUID"() -> (w4800:string)
            n3576 = local read "Serial No"() -> (w4804:string)
            n3577 = local read "Secret Key"() -> (w4805:string)
            n3578 = Concatenate Strings("\",\"MachineSerialNumber\":\"" ("string"), w4804) -> (w4808:string)
            n3579 = Concatenate Strings("\",\"ModelNumber\":\"" ("string"), w4705) -> (w4706:string)
            n3580 = Concatenate Strings("\",\"MachineRuntimeHours\":\"" ("string"), w4691) -> (w4809:string)
            n3581 = Concatenate Strings("\",\"MachineRuntimeCycles\":\"", w4700) -> (w4802:string)
            n3582 = Concatenate Strings(w4758, w4754) -> (w4788:string)
            n3583 = Concatenate Strings(w4757, w4744) -> (w4789:string)
            n3584 = Concatenate Strings(w4756, w4726) -> (w4787:string)
            n3585 = Concatenate Strings(w4808, w4706, w4809, w4802) -> (w4811:string)
            n3586 = Concatenate Strings(w4758, w4753) -> (w4785:string)
            n3587 = Concatenate Strings(w4757, w4743) -> (w4784:string)
            n3588 = Concatenate Strings(w4756, w4725) -> (w4786:string)
            n3589 = Concatenate Strings(w4758, w4752) -> (w4780:string)
            n3590 = Concatenate Strings(w4757, w4742) -> (w4781:string)
            n3591 = Concatenate Strings(w4756, w4724) -> (w4779:string)
            n3592 = Concatenate Strings(w4758, w4751) -> (w4777:string)
            n3593 = Concatenate Strings(w4757, w4741) -> (w4776:string)
            n3594 = Concatenate Strings(w4756, w4723) -> (w4778:string)
            n3595 = Concatenate Strings(w4788, w4789, w4787) -> (w4790:string)
            n3596 = Concatenate Strings(w4758, w4750) -> (w4767:string)
            n3597 = Concatenate Strings(w4757, w4740) -> (w4768:string)
            n3598 = Concatenate Strings(w4758, w4749) -> (w4764:string)
            n3599 = Concatenate Strings(w4757, w4739) -> (w4763:string)
            n3600 = Concatenate Strings(w4756, w4722) -> (w4766:string)
            n3601 = Concatenate Strings(w4756, w4721) -> (w4765:string)
            n3602 = Concatenate Strings("{\"SecretKey\":\"", w4805, w4811, "\",\"UUID\" : \"", w4800, "\",\"SensorInformation\":", "[{" ("string")) -> (w4738:string)
            n3603 = Concatenate Strings(w4785, w4784, w4786) -> (w4783:string)
            n3604 = Concatenate Strings(w4780, w4781, w4779) -> (w4782:string)
